vi "Destroy to SFTP Directory.vi"(8 "Error In":errorcluster, 10 "SFTP Attributes":refnum<class "SFTP Attributes.lvclass">, 11 "SFTP Directory In":refnum<class "SFTP Directory.lvclass">) -> (0 "Error Out":errorcluster, 3 "SFTP Directory Out":refnum<class "SFTP Directory.lvclass">)   [LabVIEW 2018, in "Toolkit.lvlib" / "SFTP Attributes.lvclass"]
uses:
  SFTP Attributes.lvclass
  SFTP Directory/SFTP Directory.lvclass
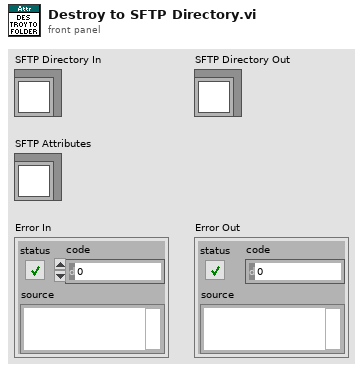
[diagram p1: front panel]
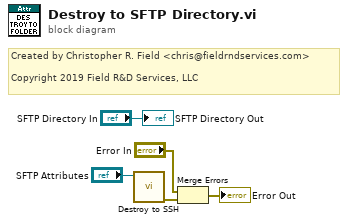
[diagram p0: block diagram]
diagram:
  # "Created by Christopher R. Field <chris@fieldrndservices.com>\n\nCopyright 2019 Field R&D Services, LLC"
  n1 = call "Destroy to SSH.vi"("SFTP Attributes"="SFTP Attributes") -> ("Error Out"=w2:errorcluster)  [unwired: 9 in, 1 out]
  n2 = Merge Errors("Error In", w2) -> (→"Error Out":errorcluster)
  "SFTP Directory Out" <- "SFTP Directory In"
